vi "MrClean.ProcEvents.vi"(0 "i ref in":refnum<vi>, 5 "error in":errorcluster) -> (14 "i ref out":refnum<vi>, 19 "error out":errorcluster)   [LabVIEW 2014, in "MrClean.lvlib"]
doc: "This method is used to define the events the object will listen to. Add your own events here."
uses:
  MrClean.lvlib
  CS_Core/BaseProcess/BaseProcess.event definition.ctl
  CS_Core/CAEObj/CAEObj.event definition.ctl
  CS_Core/BaseProcess/BaseProcess.descriptor string definition.ctl
  CS_Core/BaseProcess/BaseProcess.lvlib
  CS_Core/CAEObj/CAEObj.lvlib
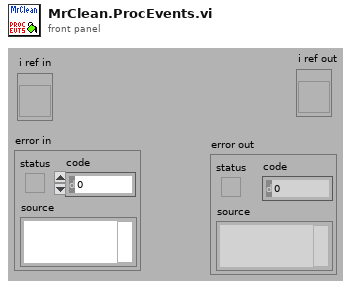
[diagram p1: front panel]
types:
  T1 = typedef "BaseProcess.lvlib/BaseProcess.event definition.ctl" = cluster{"CAEEvtDef":T2, "Data Descriptor":T3}
  T2 = typedef "CAEObj.lvlib/CAEObj.event definition.ctl" = cluster{"URL":string, "enable":bool, "ignoreResID":bool}
  T3 = typedef "BaseProcess.lvlib/BaseProcess.descriptor string definition.ctl" = string
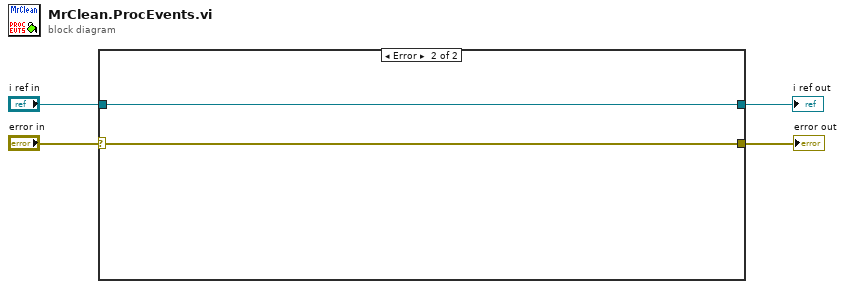
[diagram p0: block diagram]
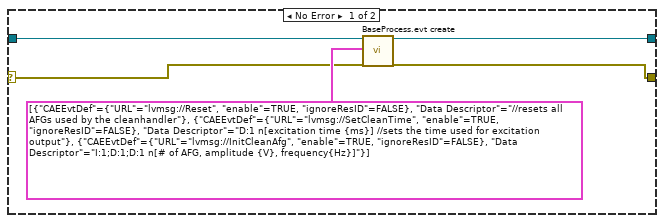
[diagram p2: hidden frame]
diagram:
  n1 = case shown="Error" "error in" {
    selector: "error in" -> [w5 w10]
    tunnel: "i ref in" -> [w9 w11]
    tunnel: [w8 w11] -> w3
    tunnel: [w7 w10] -> w2
    frame No Error {
      n2 = call "BaseProcess.evt create.vi"("i ref in"=w9, "newEvents"=T1[] [{"CAEEvtDef"={"URL"="lvmsg://Reset", "enable"=TRUE, "ignoreResID"=FALSE}, "Data Descriptor"="//resets all AFGs used by the cleanhandler"}, {"CAEEvtDef"={"URL"="lvmsg://SetCleanTime", "enable"=TRUE, "ignoreResID"=FALSE}, "Data Descriptor"="D:1 n[excitation time {ms}] //sets the time used for excitation output"}, {"CAEEvtDef"={"URL"="lvmsg://InitCleanAfg", "enable"=TRUE, "ignoreResID"=FALSE}, "Data Descriptor"="I:1;D:1;D:1 n[# of AFG, amplitude {V}, frequency{Hz}]"}] ("new events"), "error in (no error)"=w5) -> ("i ref out"=w8:refnum<vi>, "error out"=w7:errorcluster)  [unwired: 13 in, 2 out]
    }
    frame Error {
    }
  }
  "i ref out" <- w3
  "error out" <- w2
